vi "Create Actor from Template.vi"() -> ()   [LabVIEW 2020]
uses:
  <vilib>/Utility/error.llb/Error Cluster From Error Code.vi
  <vilib>/ErrorRing/Error Ring.xnode
  <resource>/Framework/Providers/MessageMakerProvider/_Message Maker/Message Maker.lvlib
  <resource>/Framework/Providers/AddActor/Add Actor.lvlib
  <vilib>/Utility/EditLVLibs/Edit LVLibs.lvlib
panel:
  out "Path Display":string caption="显示路径"
  in  "Path":path caption="保存文件至..."
  in  "Template:":string(combo) caption="模板:"
  in  "Cancel":bool
  in  "Next Button":bool
  in  "Name of Actor":string caption="操作者名"
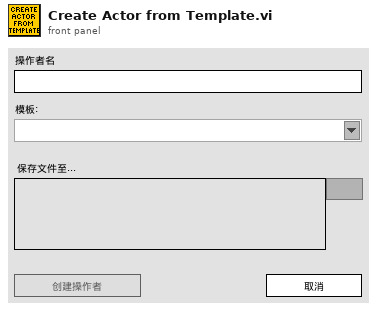
[diagram p1: front panel]
types:
  T1 = enum8{"Enabled", "Disabled", "Disabled and Grayed Out"}
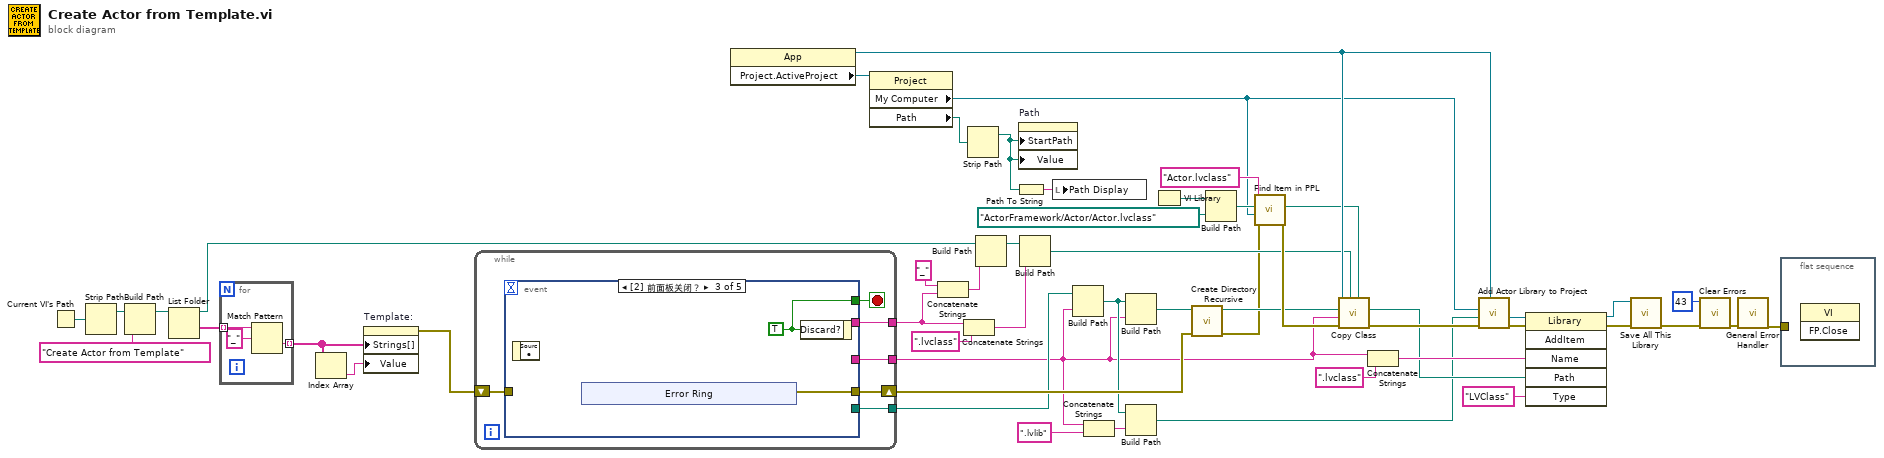
[diagram p0: block diagram]
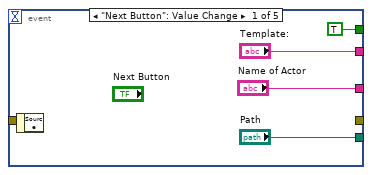
[diagram p2: hidden frame]
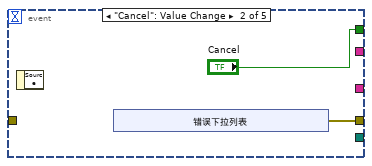
[diagram p3: hidden frame]
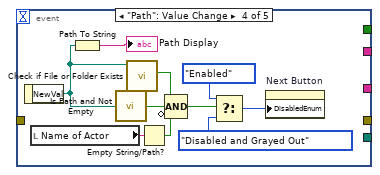
[diagram p4: hidden frame]
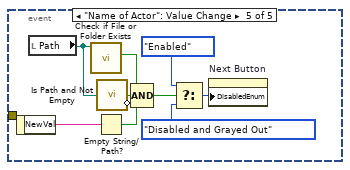
[diagram p5: hidden frame]
diagram:
  n1 = Current VI's Path() -> (path=w27:path)
  n2 = Strip Path(path=w27) -> (stripped path=w26:path)  [unwired: 1 out]
  n3 = Build Path(base path=w26, name or relative path="Create Actor from Template") -> (appended path=w13:path)
  n4 = List Folder(path=w13) -> (path out=w23:path, folder names=w17:string[])  [unwired: 3 in, 2 out]
  n5 = for {
    tunnel: w17 -> [w53] mode=indexing
    tunnel: [w52] -> w16 mode=indexing
    n6 = Match Pattern(string=w53, regular expression="_") -> (after substring=w52:string)  [unwired: 1 in, 3 out]
  }
  n7 = Index Array(array=w16) -> (element=w15:string)  [unwired: 1 in]
  n8 = property on="Template:" class="CmbBox"("Strings[]"=w16, "Value"=w15) -> (error out=w25:errorcluster)  [unwired: 2 in, 1 out]
  n9 = while {
    tunnel: [w60] -> w9
    tunnel: [w57] -> w5
    shift-right: [w59] -> w37
    shift-left: w25 -> [w58]
    tunnel: [w56] -> w11
    stop <- w55 stop-if-true
    n10 = event shown="[2] 前面板关闭？" {
      selector: _ -> [_ _ _ _ _]
      dyn-events: _ -> [_ _ _ _ _]
      timeout: _ -> [_ _ _ _ _]
      tunnel: ["Name of Actor" _ _ _ _] -> w60
      tunnel: [_ w66 w72 _ _] -> w59
      tunnel: w58 -> [_ _ _ _ _]
      tunnel: ["Template:" _ _ _ _] -> w57
      tunnel: ["Path" _ _ _ _] -> w56
      tunnel: [TRUE ("Discard?") "Cancel" w71 _ _] -> w55
      event "Next Button": Value Change {
        n11 = event-data() -> ()  [unwired: 1 in, 1 out]
      }
      event "Cancel": Value Change {
        n12 = event-data() -> ()  [unwired: 1 in, 1 out]
        n13 = xnode "错误下拉列表"() -> ("错误输出"=w66:errorcluster)
      }
      event Panel Close? {
        w71 = TRUE ("Discard?")
        n14 = event-data() -> ()  [unwired: 1 in, 1 out]
        n15 = xnode "Error Ring"() -> ("错误输出"=w72:errorcluster)
        n16 = event-data("Discard?"=w71) -> ()  [unwired: 1 in, 1 out]
      }
      event "Path": Value Change {
        n17 = event-data() -> ("NewVal"=w78:path)  [unwired: 1 in]
        n18 = local read "Name of Actor"() -> (w85:string)
        n19 = Path To String(path=w78) -> (string=→"Path Display":string)
        n20 = call <vilib>:"Is Path and Not Empty.vi"("path"=w78) -> ("Is Path and Not Empty?"=w82:bool)  [unwired: 4 in]
        n21 = call <vilib>:"Check if File or Folder Exists.vi"("path"=w78) -> ("file or folder exists?"=w84:bool)  [unwired: 8 in, 2 out]
        n22 = Empty String/Path?(string/path=w85) -> (empty?=w81:bool)
        n23 = Compound Arithmetic op=AND(w84, w82, invert w81) -> (w83:bool)
        n24 = Select(t=T1."Enabled" ("Disabled"), s=w83, f=T1."Disabled and Grayed Out" ("Disabled")) -> (s? t:f=w77:T1)
        n25 = property on="Next Button" class="Bool"("DisabledEnum"=w77) -> ()  [unwired: 2 in, 2 out]
      }
      event "Name of Actor": Value Change {
        n26 = event-data() -> ("NewVal"=w87:string)  [unwired: 1 in]
        n27 = local read "Path"() -> (w95:path)
        n28 = call <vilib>:"Check if File or Folder Exists.vi"("path"=w95) -> ("file or folder exists?"=w94:bool)  [unwired: 8 in, 2 out]
        n29 = Empty String/Path?(string/path=w87) -> (empty?=w91:bool)
        n30 = call <vilib>:"Is Path and Not Empty.vi"("path"=w95) -> ("Is Path and Not Empty?"=w92:bool)  [unwired: 4 in]
        n31 = Compound Arithmetic op=AND(w94, w92, invert w91) -> (w93:bool)
        n32 = Select(t=T1."Enabled" ("Disabled"), s=w93, f=T1."Disabled and Grayed Out" ("Disabled")) -> (s? t:f=w90:T1)
        n33 = property on="Next Button" class="Bool"("DisabledEnum"=w90) -> ()  [unwired: 2 in, 2 out]
      }
    }
  }
  n34 = property class="App"() -> (reference out=w39:refnum<vi>, "Project.ActiveProject"=w3:refnum<vi>)  [unwired: 2 in, 1 out]
  n35 = property class="Project"(reference=w3) -> ("My Computer"=w28:refnum<vi>, "Path"=w2:path)  [unwired: 1 in, 2 out]
  n36 = Concatenate Strings("_" ("regular expression"), w5) -> (w18:string)
  n37 = Concatenate Strings(w5, ".lvclass" ("regular expression")) -> (w20:string)
  n38 = Strip Path(path=w2) -> (stripped path=w1:path)  [unwired: 1 out]
  n39 = Build Path(base path=w23, name or relative path=w18) -> (appended path=w24:path)
  n40 = Path To String(path=w1) -> (string=w4:string)
  n41 = property on="Path" class="Path"("StartPath"=w1, "Value"=w1) -> ()  [unwired: 2 in, 2 out]
  n42 = Build Path(base path=w24, name or relative path=w20) -> (appended path=w22:path)
  n43 = local write "Path Display"(w4) -> ()
  n44 = Build Path(base path=w11, name or relative path=w9) -> (appended path=w10:path)
  n45 = Concatenate Strings(w9, ".lvlib" ("string")) -> (w42:string)
  n46 = Build Path(base path=w10, name or relative path=w9) -> (appended path=w8:path)
  n47 = Build Path(base path=w10, name or relative path=w42) -> (appended path=w40:path)
  n48 = VI Library() -> (path=w38:path)
  n49 = call <vilib>:"Create Directory Recursive.vi"("error in (no error)"=w37, "directory"=w8) -> ("error out"=w6:errorcluster, "directory copy"=w7:path)  [unwired: 3 in, 1 out]
  n50 = Build Path(base path=w38, name or relative path=path "ActorFramework/Actor/Actor.lvclass" ("Parent Class Path")) -> (appended path=w32:path)
  n51 = call <resource>:"Find Item in PPL.vi"("error in (no error)"=w6, "Target"=w28, "default path"=w32, "qualified name"="Actor.lvclass") -> ("error out"=w29:errorcluster, "item path out"=w31:path)  [unwired: 5 in, 1 out]
  n52 = call <resource>:"Copy Class.vi"("Parent Class Path"=w31, "Template Path"=w22, "error in (no error)"=w29, "Class Name"=w9, "Destination Directory"=w7, "AppInst"=w39) -> ("error out"=w44:errorcluster, "New Class Path"=w43:path)  [unwired: 4 in]
  n53 = Concatenate Strings(w9, ".lvclass" ("regular expression")) -> (w45:string)
  n54 = call <resource>:"Add Actor Library to Project.vi"("Application"=w39, "error in (no error)"=w44, "Library Path"=w40, "Target Item"=w28) -> ("error out"=w47:errorcluster, "Library out"=w48:refnum<vi>)  [unwired: 6 in]
  n55 = invoke class="Library" method="AddItem"(reference=w48, error in=w47, "Name"=w45, "Path"=w43, "Type"="LVClass") -> (reference out=w49:refnum<vi>, error out=w50:errorcluster)  [unwired: 1 in, 4 out]
  n56 = call <vilib>:"Save All This Library.vi"("error in (no error)"=w50, "Library in"=w49) -> ("error out"=w36:errorcluster)  [unwired: 8 in, 1 out]
  n57 = call <vilib>:"Clear Errors.vi"("error in (no error)"=w36, "specific error code to clear (0: all)"=43) -> ("error out"=w35:errorcluster)  [unwired: 4 in, 1 out]
  n58 = call <vilib>:"General Error Handler.vi"("error in (no error)"=w35) -> ("error out"=w14:errorcluster)  [unwired: 10 in, 4 out]
  n59 = flat-sequence {
    tunnel: w14 -> [_]
    frame #0 {
      n60 = invoke class="VI" method="FP.Close"() -> ()  [unwired: 3 in, 3 out]
    }
  }
